vi "HIN.vi"(0 "System no.":i32=1 min=1 max=4 step=1, 2 "Axes to command":string[](array[string]), 3 "HID control":bool[](array[boolean]), 5 "error in":errorcluster) -> (19 "error out":errorcluster)   [LabVIEW 2026]
doc: "Activates or deactivates HID control for given axes of the controller. See controller user manual for details.\n\nC-867:"
panel:
  # "Activates or deactivates HID control for given axes of the \ncontroller. See controller User Manual for details."
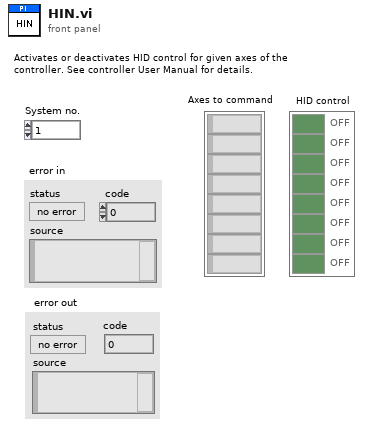
[diagram p1: front panel]
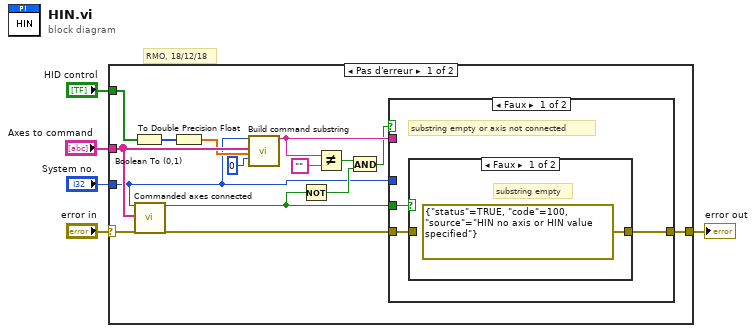
[diagram p0: block diagram]
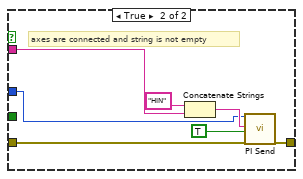
[diagram p3: hidden frame]
diagram:
  # "RMO, 18/12/18"
  n1 = case shown="Pas d'erreur" "error in" {
    selector: "error in" -> [w6 w33]
    tunnel: [w20 w33] -> w5
    tunnel: "System no." -> [w8 _]
    tunnel: "Axes to command" -> [w16 _]
    tunnel: "HID control" -> [w11 _]
    frame No Error {
      n2 = Boolean To (0,1)(Boolean=w11) -> (0, 1=w10:i16[])
      n3 = call "Commanded axes connected.vi"("System no."=w8, "Commanded axes"=w16, "error in"=w6) -> ("Controller error"=w14:bool, "error out"=w17:errorcluster)  [unwired: 1 in, 14 out]
      n4 = To Double Precision Float(number=w10) -> (double precision float=w9:dbl[])
      n5 = call "Build command substring.vi"("System no."=w8, "Affected axes"=w16, "Parameters"=w9, "No. of digits"=i16 0 ("No.of digits")) -> ("Command substring"=w18:string)  [unwired: 3 in, 12 out]
      n6 = Not(x=w14) -> (.not. x?=w13:bool)
      n7 = Not Equal?(x=w18, y="") -> (x != y?=w15:bool)
      n8 = And(x=w15, y=w13) -> (x .and. y?=w12:bool)
      n9 = case shown="Faux" w12 {
        tunnel: w18 -> [_ w31]
        tunnel: [w23 w27] -> w20
        tunnel: w17 -> [w21 w28]
        tunnel: w14 -> [w22 _]
        tunnel: w8 -> [_ w26]
        frame False {
          # "substring empty or axis not connected"
          n10 = case shown="Faux" w22 {
            tunnel: [errorcluster {"status"=TRUE, "code"=100, "source"="HIN no axis or HIN value specified"} ("error out") w25] -> w23
            tunnel: w21 -> [_ w25]
            frame False {
              # "substring empty"
            }
            frame True {
              # "commanded axis not connected"
            }
          }
        }
        frame True {
          # "axes are connected and string is not empty"
          n11 = Concatenate Strings("HIN", w31) -> (w29:string)
          n12 = call "PI Send.vi"("System no."=w26, "String to send"=w29, "Attach termination char.?"=TRUE ("Attach Linefeed?"), "error in"=w28) -> ("error out"=w27:errorcluster)  [unwired: 2 in, 13 out]
        }
      }
    }
    frame Error {
    }
  }
  "error out" <- w5
